vi "Release Gate Reference.vi"(8 "error in (no error)":errorcluster, 9 "force destroy? (F)":bool, 11 "gate":T1) -> (0 "error out":errorcluster, 3 "gate name":string)   [LabVIEW 2015, in "Gates.lvlib"]
doc: "Releases a reference to a gate."
uses:
  Gates.lvlib
  Gate.ctl
  Gate Pass.ctl
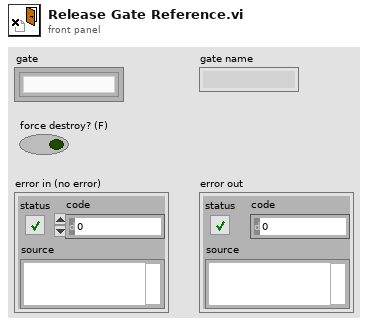
[diagram p1: front panel]
types:
  T1 = typedef "Gates.lvlib/Gate.ctl" = refnum<k1>
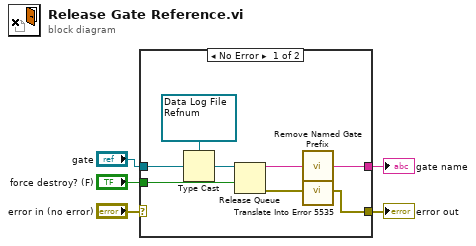
[diagram p0: block diagram]
diagram:
  n1 = case shown="No Error" "error in (no error)" {
    selector: "error in (no error)" -> [_ w14]
    tunnel: "force destroy? (F)" -> [w13 _]
    tunnel: "gate" -> [w11 _]
    tunnel: [w8 _] -> w3
    tunnel: [w6 w14] -> w1
    frame No Error {
      w10 = refnum<queue> refnum items=["Gate Pass"] ("queue out")
      n2 = Type Cast(type=w10, x=w11) -> (*(type *) &x=w12:refnum<queue>)
      n3 = Release Queue(queue=w12, force destroy? (F)=w13) -> (queue name=w9:string, error out=w7:errorcluster)  [unwired: 1 in, 1 out]
      n4 = call "Remove Named Gate Prefix.vi"("name in"=w9) -> ("name out"=w8:string)
      n5 = call "Translate Into Error 5535.vi"("error in (no error)"=w7) -> ("error out"=w6:errorcluster)  [unwired: 1 in]
    }
    frame Error {
    }
  }
  "error out" <- w1
  "gate name" <- w3
